vi "Build sensor path.vi"(3 "error in":errorcluster) -> (7 "Current test directory":path, 10 "error out":errorcluster)   [LabVIEW 2018]
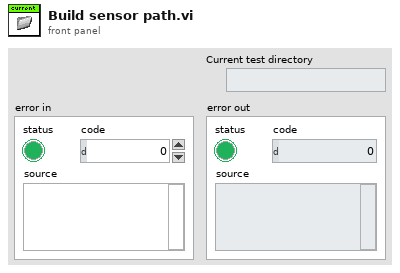
[diagram p1: front panel]
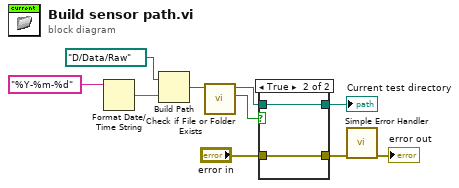
[diagram p0: block diagram]
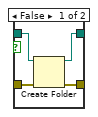
[diagram p2: hidden frame]
diagram:
  n1 = Format Date/Time String(time format string (%c)="%Y-%m-%d") -> (date/time string=w8:string)  [unwired: 2 in]
  n2 = Build Path(base path=path "D:/Data/Raw", name or relative path=w8) -> (appended path=w3:path)
  n3 = call <vilib>:"Check if File or Folder Exists.vi"("path"=w3) -> ("file or folder exists?"=w9:bool, "dup path"=w10:path)  [unwired: 8 in, 1 out]
  n4 = case shown="True" w9 {
    tunnel: w10 -> [w14 w16]
    tunnel: [w13 w16] -> w2
    tunnel: "error in" -> [w12 w15]
    tunnel: [w11 w15] -> w1
    frame False {
      n5 = Create Folder(path (use dialog)=w14, error in=w12) -> (created path=w13:path, error out=w11:errorcluster)  [unwired: 1 in, 1 out]
    }
    frame True {
    }
  }
  "Current test directory" <- w2
  n6 = call <vilib>:"Simple Error Handler.vi"("error in (no error)"=w1) -> ("error out"=→"error out":errorcluster)  [unwired: 4 in, 4 out]
